vi "Slider (Main).vi"(6 "Playback":bool, 8 "Slider":i16(slide) scale=0.0..10.0, 10 "Stop":bool, 11 "Error in":errorcluster) -> (15 "Error out":errorcluster)   [LabVIEW 2020]
doc: "This system is used to playback the previous data which is needed to be plotted in the chart and the current value will also be plotted"
uses:
  Typedefs/Cluster data.ctl
panel:
  # "Dynamic and User Events"
  # "Click this button to play the previous value \nrecorded"
  # "Click this button to stop the execution of the VI"
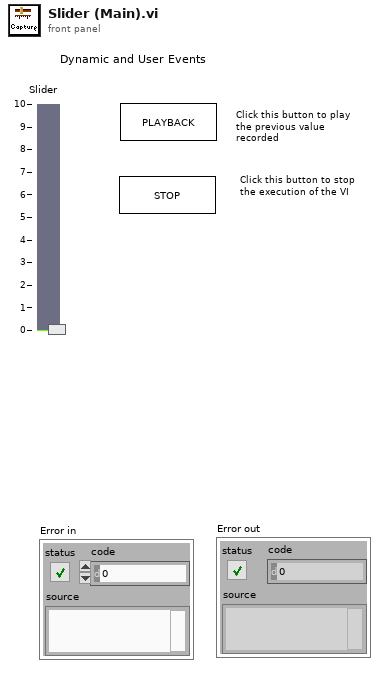
[diagram p1: front panel]
types:
  T1 = enum16{"Get Ref", "Destroy", "Create", "Generate"}
  T2 = typedef "Cluster data.ctl" = cluster{"Position":dbl, "Delay":dbl, "Boolean":bool}
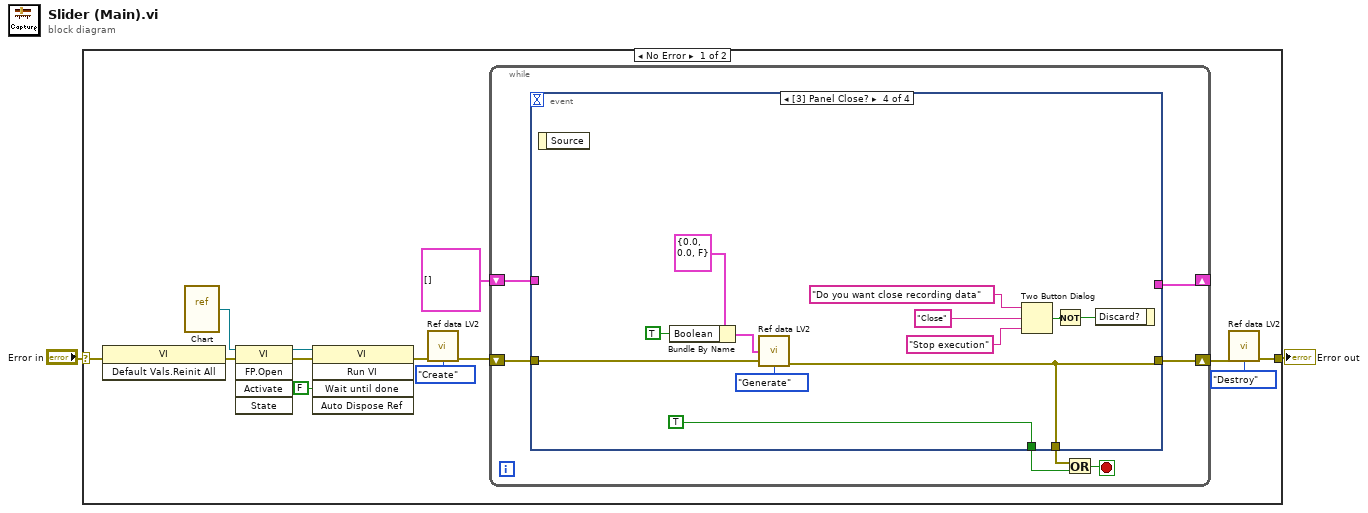
[diagram p0: block diagram]
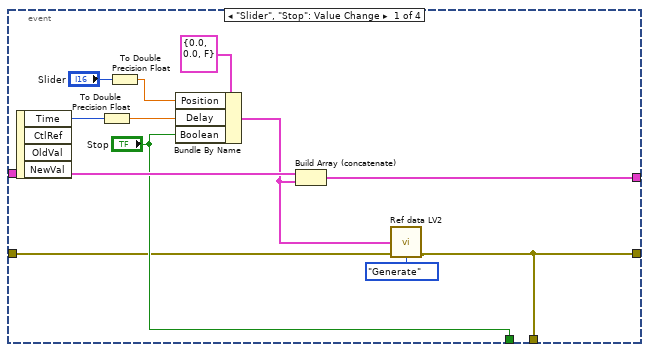
[diagram p2: hidden frame]
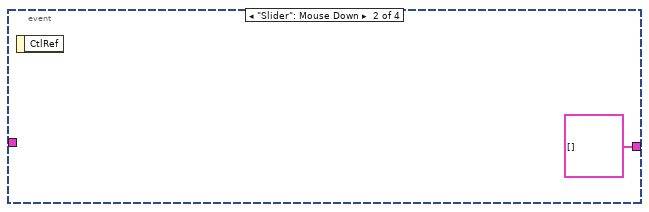
[diagram p3: hidden frame]
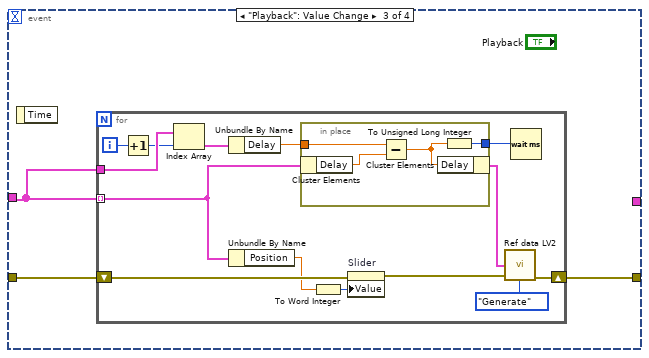
[diagram p4: hidden frame]
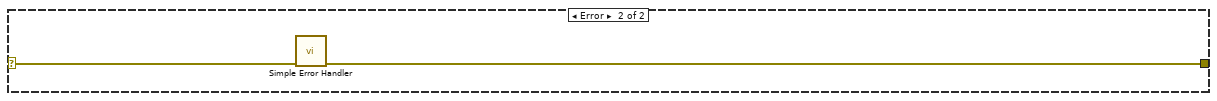
[diagram p5: hidden frame]
diagram:
  n1 = case shown="No Error" "Error in" {
    selector: "Error in" -> [w13 w70]
    tunnel: [w6 w69] -> w1
    frame No Error {
      n2 = invoke class="VI" method="Default Vals.Reinit All"(error in=w13) -> (error out=w11:errorcluster)  [unwired: 2 in, 2 out]
      n3 = vi-ref "Chart.vi"() -> (w8:refnum<vi>)
      n4 = invoke class="VI" method="FP.Open"(reference=w8, error in=w11) -> (reference out=w10:refnum<vi>, error out=w9:errorcluster)  [unwired: 3 in, 3 out]
      n5 = invoke class="VI" method="Run VI"(reference=w10, error in=w9, "Wait until done"=FALSE ("Wait Until Done")) -> (error out=w12:errorcluster)  [unwired: 2 in, 4 out]
      n6 = call "Ref data LV2.vi"("error in"=w12, "Enum"=T1."Create") -> ("error out"=w7:errorcluster)  [unwired: 12 in, 1 out]
      n7 = while {
        shift-right: [w21] -> w5
        shift-left: w7 -> [w22]
        shift-right: [w19] -> _
        shift-left: T2[] [] -> [w18]
        stop <- w20 stop-if-true
        n8 = event shown="[3] Panel Close?" {
          selector: _ -> [_ _ _ _]
          dyn-events: _ -> [_ _ _ _]
          timeout: _ -> [_ _ _ _]
          tunnel: [w26 _ w36 w58] -> w21
          tunnel: w22 -> [w27 _ w37 w59]
          tunnel: [w34 T2[] [] _ _] -> w19
          tunnel: w18 -> [w33 _ w38 _]
          tunnel: [w26 _ _ w58] -> w17
          tunnel: ["Stop" _ _ TRUE] -> w16
          event "Slider", "Stop": Value Change {
            n9 = event-data() -> ("Time"=w30:u32)  [unwired: 1 in, 3 out]
            n10 = To Double Precision Float(number=w30) -> (double precision float=w24:dbl)
            n11 = To Double Precision Float(number="Slider") -> (double precision float=w23:dbl)
            n12 = Bundle By Name(cluster=T2 {"Position"=0.0, "Delay"=0.0, "Boolean"=FALSE} ("Data"), "Position"=w23, "Delay"=w24, "Boolean"="Stop") -> (w25:T2)
            n13 = Build Array (concatenate)(w33, w25) -> (w34:T2[])
            n14 = call "Ref data LV2.vi"("Data"=w25, "error in"=w27, "Enum"=T1."Generate") -> ("error out"=w26:errorcluster)  [unwired: 11 in, 1 out]
          }
          event "Slider": Mouse Down {
            n15 = event-data() -> ()  [unwired: 1 in, 1 out]
          }
          event "Playback": Value Change {
            n16 = event-data() -> ()  [unwired: 1 in, 1 out]
            n17 = for {
              tunnel: w38 -> [w49] mode=indexing
              tunnel: w38 -> [w51]
              shift-right: [w47] -> w36
              shift-left: w37 -> [w48]
              i -> [w52]
              n18 = Increment(x=w52) -> (x+1=w50:i32)
              n19 = Index Array(array=w51, index=w50) -> (element=w46:T2)
              n20 = Unbundle By Name(w46) -> ("Delay"=w45:dbl)
              n21 = Unbundle By Name(w49) -> ("Position"=w41:dbl)
              n22 = in-place {
                in-place-border: w45 -> [w56]
                in-place-border: [w53] -> w39
                n23 = in-place-cluster #1(w49) -> ("Delay"=w55:dbl)
                n24 = Subtract(x=w56, y=w55) -> (x-y=w54:dbl)
                n25 = in-place-cluster #1("Delay"=w54) -> (w44:T2)
                n26 = To Unsigned Long Integer(number=w54) -> (unsigned 32bit integer=w53:u32)
              }
              n27 = To Word Integer(number=w41) -> (16bit integer=w42:i16)
              n28 = property on="Slider" class="Slide (strict)"(error in=w48, "Value"=w42) -> (error out=w40:errorcluster)  [unwired: 1 in, 1 out]
              n29 = call "Ref data LV2.vi"("Data"=w44, "error in"=w40, "Enum"=T1."Generate") -> ("error out"=w47:errorcluster)  [unwired: 11 in, 1 out]
              n30 = Wait (ms)(milliseconds to wait=w39) -> ()  [unwired: 1 out]
            }
          }
          event Panel Close? {
            n31 = event-data() -> ()  [unwired: 1 in, 1 out]
            n32 = Bundle By Name(cluster=T2 {"Position"=0.0, "Delay"=0.0, "Boolean"=FALSE} ("Data"), "Boolean"=TRUE) -> (w57:T2)
            n33 = call "Ref data LV2.vi"("Data"=w57, "error in"=w59, "Enum"=T1."Generate") -> ("error out"=w58:errorcluster)  [unwired: 11 in, 1 out]
            n34 = Two Button Dialog(message="Do you want close recording data", 1:"Stop execution" ("F button name (\"Cancel\")"), 2:"Close" ("T button name (\"OK\")")) -> (T button?=w64:bool)
            n35 = Not(x=w64) -> (.not. x?=w65:bool)
            n36 = event-data("Discard?"=w65) -> ()  [unwired: 1 in, 1 out]
          }
        }
        n37 = Or(x=w17, y=w16) -> (x .or. y?=w20:bool)
      }
      n38 = call "Ref data LV2.vi"("error in"=w5, "Enum"=T1."Destroy") -> ("error out"=w6:errorcluster)  [unwired: 12 in, 1 out]
    }
    frame Error {
      n39 = call <vilib>:"Simple Error Handler.vi"("error in (no error)"=w70) -> ("error out"=w69:errorcluster)  [unwired: 4 in, 4 out]
    }
  }
  "Error out" <- w1
